vi "Check Nim update file for unique esim.vi"() -> ()   [LabVIEW 2013]
uses:
  <vilib>/Utility/file.llb/Read From Spreadsheet File (string).vi
panel:
  out "Got dups?":bool
  out "all rows":string[][](array[string])
  out "test sim id":string[](array[string])
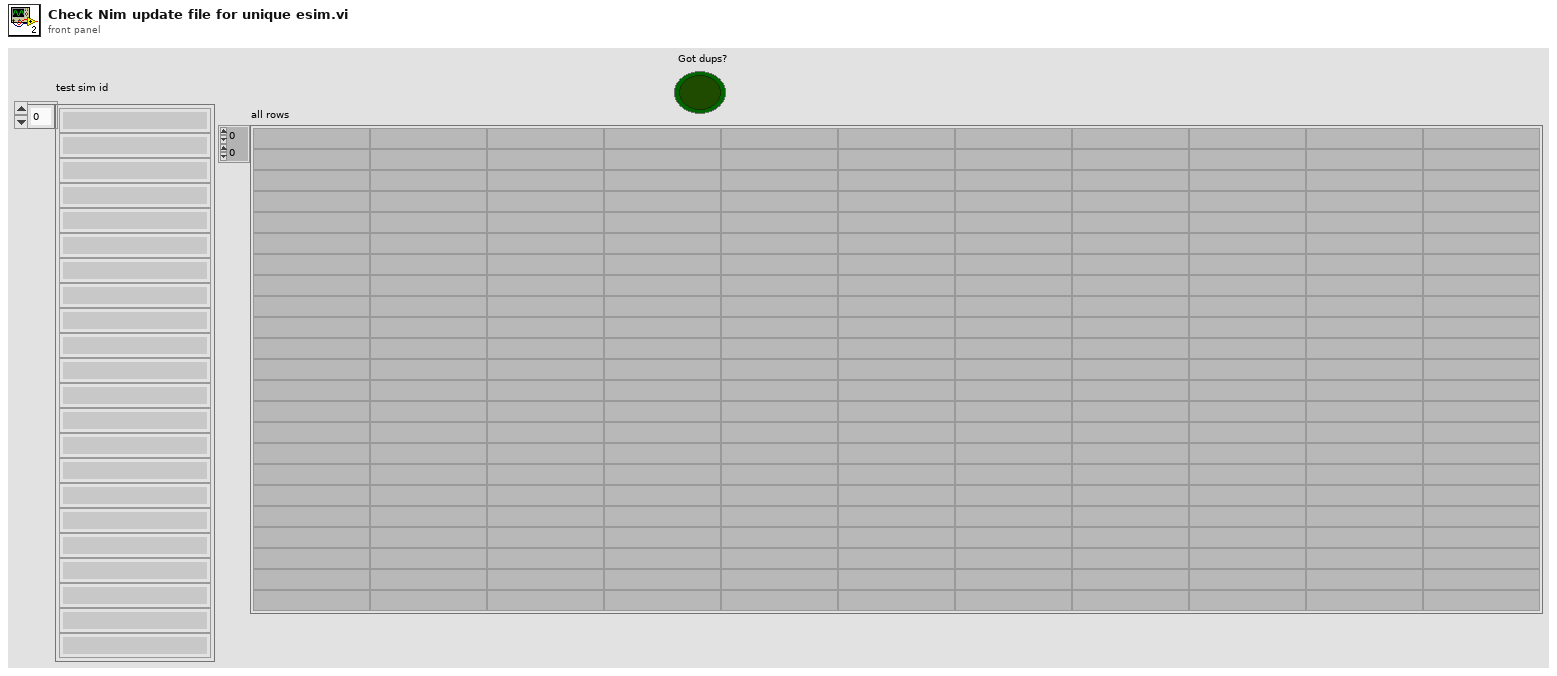
[diagram p1: front panel]
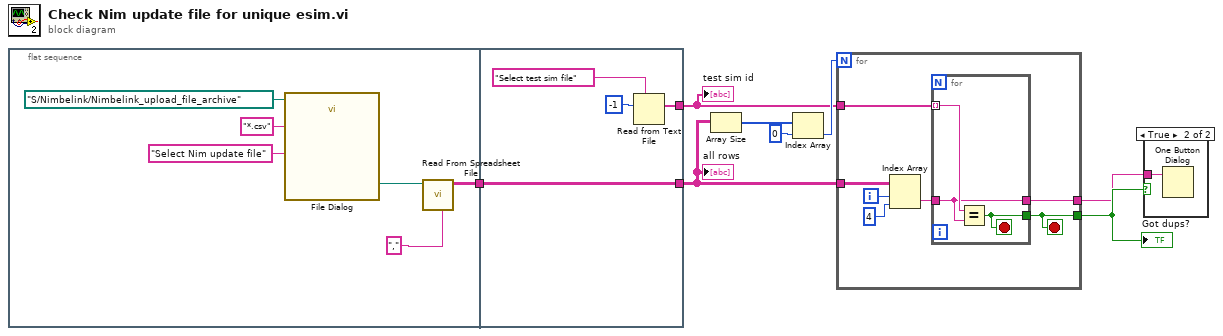
[diagram p0: block diagram]
diagram:
  n1 = flat-sequence {
    tunnel: [w13] -> w2
    tunnel: [w18] -> w5
    tunnel: w2 -> [w18]
    tunnel: [w15] -> w1
    frame #0 {
      n2 = call "File Dialog"("start path"=path "S:/Nimbelink/Nimbelink_upload_file_archive", "prompt"="Select Nim update file", "pattern (all files)"="*.csv") -> ("selected path"=w9:path)  [unwired: 9 in, 3 out]
      n3 = call-poly <vilib>:"Read From Spreadsheet File.vi"("delimiter (\\t)"="," ("delimiter (\\t)"), "file path (dialog if empty)"=w9) -> ("all rows"=w13:string[][])  [unwired: 5 in, 4 out]
    }
    frame #1 {
      n4 = Read from Text File(prompt (Open existing file)="Select test sim file", count=-1) -> (text=w15:string[])  [unwired: 2 in, 3 out]
    }
  }
  n5 = Array Size(array=w5) -> (size(s)=w8:i32[])
  n6 = Index Array(array=w8, index=0) -> (element=w6:i32)
  n7 = for {
    N: w6 -> [_]
    tunnel: w5 -> [w25]
    tunnel: w1 -> [w22]
    tunnel: [w20] -> w4
    tunnel: [w19] -> w3
    i -> [w24]
    stop <- w20 stop-if-true
    n8 = Index Array(array=w25, index (row)=w24, index (col)=4 ("disabled index (col)")) -> (element=w21:string)
    n9 = for {
      tunnel: w22 -> [w28] mode=indexing
      tunnel: w21 -> [w26]
      tunnel: [w27] -> w20
      tunnel: [w26] -> w19
      stop <- w27 stop-if-true
      n10 = Equal?(x=w28, y=w26) -> (x = y?=w27:bool)
    }
  }
  "Got dups?" <- w4
  n11 = case shown="True" w4 {
    tunnel: w3 -> [_ w29]
    frame False {
    }
    frame True {
      n12 = One Button Dialog(message=w29) -> ()  [unwired: 1 in, 1 out]
    }
  }
  "test sim id" <- w1
  "all rows" <- w5
